vi "gentec-M-Link.Get Trigger Level.vi"(0 "VISA resource In":refnum<visa-resource-name>, 5 "error in (no error)":errorcluster) -> (11 "Data Read":string, 13 "Read Timeout":bool, 14 "VISA resource Out":refnum<visa-resource-name>, 16 "Trigger Level [%]":dbl, 17 "Error":bool, 19 "error out":errorcluster)   [LabVIEW 2014, in "gentec-M-Link - Driver.lvlib"]
doc: "Data to write: trg\n\nQueries the instrument trigger level. Returns the trigger level in percent."
uses:
  gentec-M-Link - Driver.lvlib
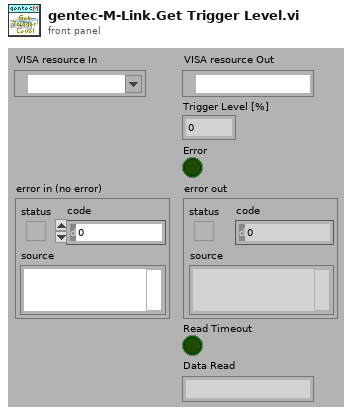
[diagram p1: front panel]
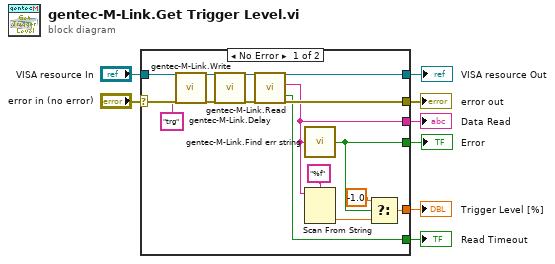
[diagram p0: block diagram]
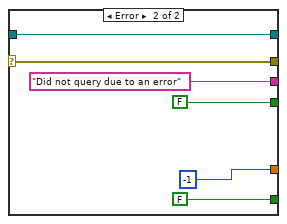
[diagram p2: hidden frame]
diagram:
  n1 = case shown="No Error" "error in (no error)" {
    selector: "error in (no error)" -> [w21 w30]
    tunnel: [w22 w30] -> w7
    tunnel: "VISA resource In" -> [w20 w29]
    tunnel: [w19 w29] -> w5
    tunnel: [w10 -1] -> w4
    tunnel: [w13 "Did not query due to an error" ("Data Read")] -> w3
    tunnel: [w14 FALSE ("Read Timeout")] -> w2
    tunnel: [w12 FALSE ("Found")] -> w1
    frame No Error {
      n2 = call "gentec-M-Link.Write.vi"("VISA resource (In)"=w20, "Data To Write"="trg" ("format string"), "error in (no error)"=w21) -> ("VISA resource (Out)"=w24:refnum<visa-resource-name>, "error out"=w23:errorcluster)  [unwired: 14 in, 1 out]
      n3 = call "gentec-M-Link.Delay.vi"("VISA resource In"=w24, "error in (no error)"=w23) -> ("VISA resource Out"=w18:refnum<visa-resource-name>, "error out"=w17:errorcluster)  [unwired: 16 in]
      n4 = call "gentec-M-Link.Read.vi"("VISA resource (In)"=w18, "error in (no error)"=w17) -> ("VISA resource (Out)"=w19:refnum<visa-resource-name>, "Data Read"=w13:string, "Read Timeout"=w14:bool, "error out"=w22:errorcluster)  [unwired: 13 in, 1 out]
      n5 = call "gentec-M-Link.Find err string.vi"("string"=w13) -> ("Found"=w12:bool)
      n6 = Scan From String(format string="%f", input string=w13) -> (output 1=w11:dbl)  [unwired: 3 in, 3 out]
      n7 = Select(t=-1.0, s=w12, f=w11) -> (s? t:f=w10:dbl)
    }
    frame Error {
    }
  }
  "error out" <- w7
  "VISA resource Out" <- w5
  "Trigger Level [%]" <- w4
  "Data Read" <- w3
  "Read Timeout" <- w2
  "Error" <- w1
